vi "string to digital waveform.vi"(1 "String":string) -> (0 "digital waveform":digitalwaveform(waveform))   [LabVIEW 2009]
uses:
  <vilib>/Waveform/DWDTOps.llb/DWDT Binary U8 to Digital.vi
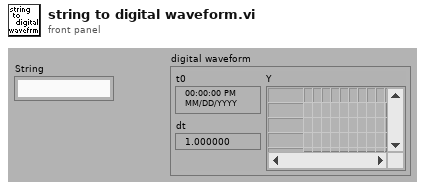
[diagram p1: front panel]
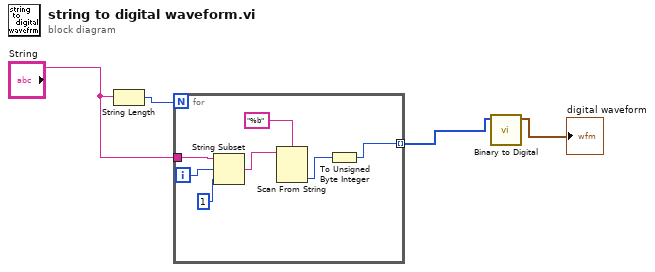
[diagram p0: block diagram]
diagram:
  n1 = String Length(string="String") -> (length=w1:i32)
  n2 = for {
    N: w1 -> [_]
    tunnel: "String" -> [w8]
    tunnel: [w5] -> w3 mode=indexing
    i -> [w9]
    n3 = String Subset(string=w8, offset (0)=w9, length (rest)=1 ("length (rest)")) -> (substring=w7:string)
    n4 = Scan From String(format string="%b", input string=w7) -> (output 1=w6:i32)  [unwired: 2 in, 4 out]
    n5 = To Unsigned Byte Integer(number=w6) -> (unsigned 8bit integer=w5:u8)
  }
  n6 = call-poly <vilib>:"Binary to Digital.vi"("binary array"=w3) -> ("digital waveform"=→"digital waveform":digitalwaveform)  [unwired: 3 in, 7 out]
